vi "Preset subsystems.vi"(11 "Enum":T1(ring)) -> ()   [LabVIEW 2018]
uses:
  f200bb85-f6e8-4092-baee-461cfbd7f02f.vi
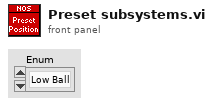
[diagram p1: front panel]
types:
  T1 = enum16{"Low Ball", "Middle Ball", "High Ball", "High Hatch", "Middle Hatch", "Low Hatch", "Cargo Ball", "Ball Loading Station", "Ball Ground", "Reserve"}
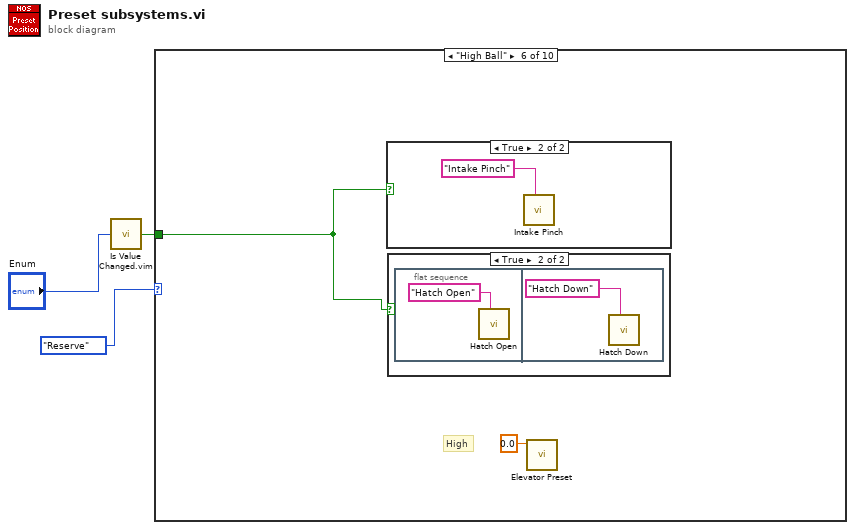
[diagram p0: block diagram]
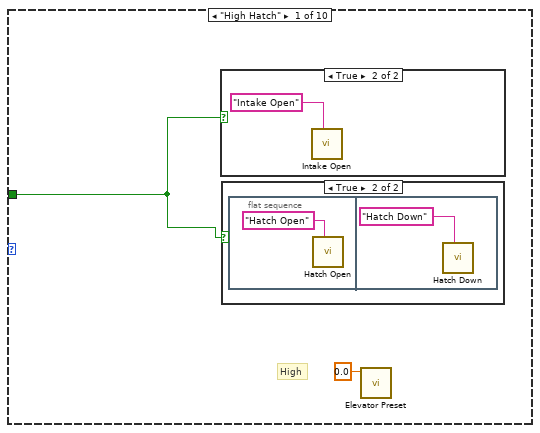
[diagram p2: hidden frame]
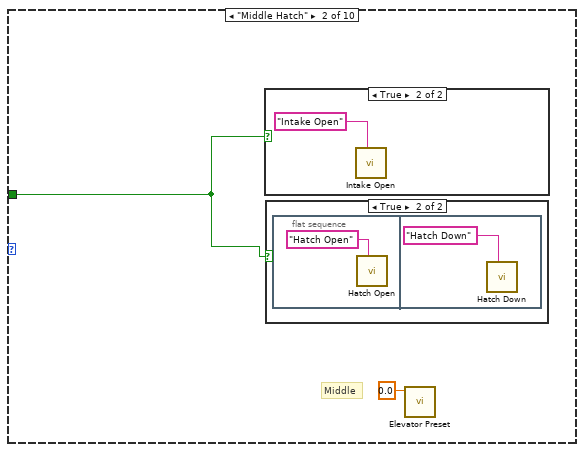
[diagram p5: hidden frame]
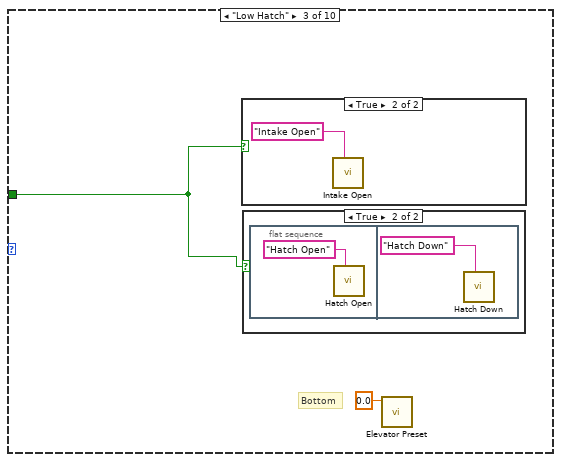
[diagram p8: hidden frame]
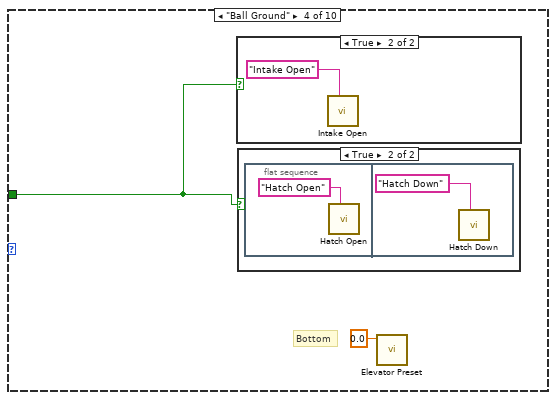
[diagram p11: hidden frame]
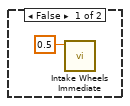
[diagram p12: hidden frame]
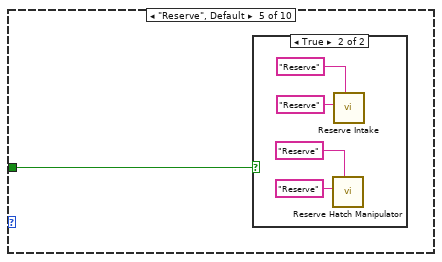
[diagram p14: hidden frame]
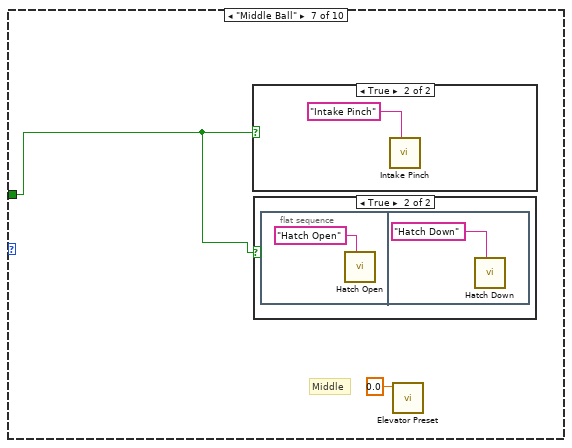
[diagram p18: hidden frame]
diagram:
  n1 = call "Is Value Changed.vim"("value"="Enum") -> ("changed or first call?"=w2:bool)
  n2 = case shown="\"High Ball\"" T1."Reserve" ("Enum") {
    tunnel: w2 -> [w4 w9 w14 w19 w25 w30 w35 w40 _ _]
    frame "High Hatch" {
      # "High"
      n3 = case shown="True" w4 {
        frame False {
        }
        frame True {
          n4 = call "Intake Open.vi"("Description"="Intake Open") -> ()  [unwired: 10 in, 1 out]
        }
      }
      n5 = case shown="True" w4 {
        frame False {
        }
        frame True {
          n6 = flat-sequence {
            frame #0 {
              n7 = call "Hatch Open.vi"("Description"="Hatch Open") -> ()  [unwired: 10 in, 1 out]
            }
            frame #1 {
              n8 = call "Hatch Down.vi"("Description"="Hatch Down") -> ()  [unwired: 10 in, 1 out]
            }
          }
        }
      }
      n9 = call "Elevator Preset.vi"("Position"=0.0) -> ()  [unwired: 10 in, 1 out]
    }
    frame "Middle Hatch" {
      # "Middle"
      n10 = case shown="True" w9 {
        frame False {
        }
        frame True {
          n11 = call "Intake Open.vi"("Description"="Intake Open") -> ()  [unwired: 10 in, 1 out]
        }
      }
      n12 = case shown="True" w9 {
        frame False {
        }
        frame True {
          n13 = flat-sequence {
            frame #0 {
              n14 = call "Hatch Open.vi"("Description"="Hatch Open") -> ()  [unwired: 10 in, 1 out]
            }
            frame #1 {
              n15 = call "Hatch Down.vi"("Description"="Hatch Down") -> ()  [unwired: 10 in, 1 out]
            }
          }
        }
      }
      n16 = call "Elevator Preset.vi"("Position"=0.0) -> ()  [unwired: 10 in, 1 out]
    }
    frame "Low Hatch" {
      # "Bottom"
      n17 = case shown="True" w14 {
        frame False {
        }
        frame True {
          n18 = call "Intake Open.vi"("Description"="Intake Open") -> ()  [unwired: 10 in, 1 out]
        }
      }
      n19 = case shown="True" w14 {
        frame False {
        }
        frame True {
          n20 = flat-sequence {
            frame #0 {
              n21 = call "Hatch Open.vi"("Description"="Hatch Open") -> ()  [unwired: 10 in, 1 out]
            }
            frame #1 {
              n22 = call "Hatch Down.vi"("Description"="Hatch Down") -> ()  [unwired: 10 in, 1 out]
            }
          }
        }
      }
      n23 = call "Elevator Preset.vi"("Position"=0.0) -> ()  [unwired: 10 in, 1 out]
    }
    frame "Ball Ground" {
      # "Bottom"
      n24 = case shown="True" w19 {
        frame False {
          n25 = call "Intake Wheels Immediate.vi"("Setpoint"=0.5) -> ()  [unwired: 10 in, 1 out]
        }
        frame True {
          n26 = call "Intake Open.vi"("Description"="Intake Open") -> ()  [unwired: 10 in, 1 out]
        }
      }
      n27 = case shown="True" w19 {
        frame False {
        }
        frame True {
          n28 = flat-sequence {
            frame #0 {
              n29 = call "Hatch Open.vi"("Description"="Hatch Open") -> ()  [unwired: 10 in, 1 out]
            }
            frame #1 {
              n30 = call "Hatch Down.vi"("Description"="Hatch Down") -> ()  [unwired: 10 in, 1 out]
            }
          }
        }
      }
      n31 = call "Elevator Preset.vi"("Position"=0.0) -> ()  [unwired: 10 in, 1 out]
    }
    frame "Reserve", Default {
      n32 = case shown="True" w25 {
        frame False {
        }
        frame True {
          n33 = call "Reserve Hatch Manipulator.vi"("Description"="Reserve", "Command Name"="Reserve") -> ()  [unwired: 9 in, 1 out]
          n34 = call "Reserve Intake.vi"("Description"="Reserve", "Command Name"="Reserve") -> ()  [unwired: 9 in, 1 out]
        }
      }
    }
    frame "High Ball" {
      # "High"
      n35 = case shown="True" w30 {
        frame False {
        }
        frame True {
          n36 = call "Intake Pinch.vi"("Description"="Intake Pinch") -> ()  [unwired: 10 in, 1 out]
        }
      }
      n37 = case shown="True" w30 {
        frame False {
        }
        frame True {
          n38 = flat-sequence {
            frame #0 {
              n39 = call "Hatch Open.vi"("Description"="Hatch Open") -> ()  [unwired: 10 in, 1 out]
            }
            frame #1 {
              n40 = call "Hatch Down.vi"("Description"="Hatch Down") -> ()  [unwired: 10 in, 1 out]
            }
          }
        }
      }
      n41 = call "Elevator Preset.vi"("Position"=0.0) -> ()  [unwired: 10 in, 1 out]
    }
    frame "Middle Ball" {
      # "Middle"
      n42 = case shown="True" w35 {
        frame False {
        }
        frame True {
          n43 = call "Intake Pinch.vi"("Description"="Intake Pinch") -> ()  [unwired: 10 in, 1 out]
        }
      }
      n44 = case shown="True" w35 {
        frame False {
        }
        frame True {
          n45 = flat-sequence {
            frame #0 {
              n46 = call "Hatch Open.vi"("Description"="Hatch Open") -> ()  [unwired: 10 in, 1 out]
            }
            frame #1 {
              n47 = call "Hatch Down.vi"("Description"="Hatch Down") -> ()  [unwired: 10 in, 1 out]
            }
          }
        }
      }
      n48 = call "Elevator Preset.vi"("Position"=0.0) -> ()  [unwired: 10 in, 1 out]
    }
    frame "Low Ball" {
      # "Bottom"
      n49 = case shown="True" w40 {
        frame False {
        }
        frame True {
          n50 = call "Intake Pinch.vi"("Description"="Intake Pinch") -> ()  [unwired: 10 in, 1 out]
        }
      }
      n51 = case shown="True" w40 {
        frame False {
        }
        frame True {
          n52 = flat-sequence {
            frame #0 {
              n53 = call "Hatch Open.vi"("Description"="Hatch Open") -> ()  [unwired: 10 in, 1 out]
            }
            frame #1 {
              n54 = call "Hatch Down.vi"("Description"="Hatch Down") -> ()  [unwired: 10 in, 1 out]
            }
          }
        }
      }
      n55 = call "Elevator Preset.vi"("Position"=0.0) -> ()  [unwired: 10 in, 1 out]
    }
    frame "Cargo Ball" {
    }
    frame "Ball Loading Station" {
    }
  }
